vi "RichToFlatni_measurementlink_sessionmanagement_v1_GetMultiplexerSessionsRequest.vi"(5 "OutputClusterType":T1, 11 "InputCluster":T3) -> (3 "OutputCluster":T1)   [LabVIEW 2020, in "MeasurementLink Session Management Client.lvlib"]
uses:
  MeasurementLink Session Management Client.lvlib
  ni_measurementlink_sessionmanagement_v1_GetMultiplexerSessionsRequest.ctl
  ni_measurementlink_PinMapContext.ctl
  ni_measurementlink_sessionmanagement_v1_GetMultiplexerSessionsRequest_Flat.ctl
  ni_measurementlink_PinMapContext_Flat.ctl
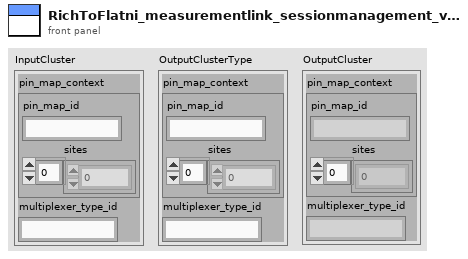
[diagram p1: front panel]
types:
  T1 = typedef "MeasurementLink Session Management Client.lvlib/ni_measurementlink_sessionmanagement_v1_GetMultiplexerSessionsRequest_Flat.ctl" = cluster{"pin_map_context":T2, "multiplexer_type_id":string}
  T2 = typedef "MeasurementLink Session Management Client.lvlib/ni_measurementlink_PinMapContext_Flat.ctl" = cluster{"pin_map_id":string, "sites":i32[]}
  T3 = typedef "MeasurementLink Session Management Client.lvlib/ni_measurementlink_sessionmanagement_v1_GetMultiplexerSessionsRequest.ctl" = cluster{"pin_map_context":T4, "multiplexer_type_id":string}
  T4 = typedef "MeasurementLink Session Management Client.lvlib/ni_measurementlink_PinMapContext.ctl" = cluster{"pin_map_id":string, "sites":i32[]}
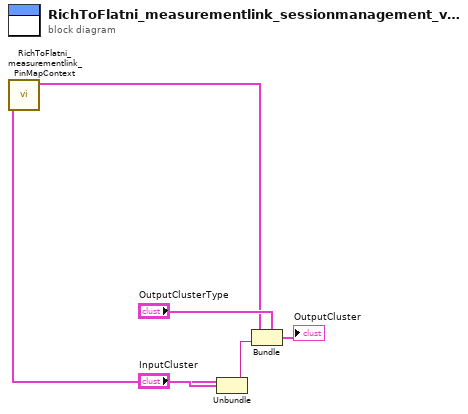
[diagram p0: block diagram]
diagram:
  n1 = Unbundle "Unbundle"("InputCluster") -> ("pin_map_context"=w3:T4, "multiplexer_type_id"=w1:string)
  n2 = call "RichToFlatni_measurementlink_PinMapContext.vi"("InputCluster"=w3) -> ("OutputCluster"=w2:T2)  [unwired: 10 in]
  n3 = Bundle "Bundle"(cluster="OutputClusterType", "pin_map_context"=w2, "multiplexer_type_id"=w1) -> (→"OutputCluster":T1)
